vi "4145 Set GUI controls.vi"(0 "Simple/Advanced Checked?":bool, 5 "Panel Controls[]":refnum<vi>[](array[refnum]), 7 "X axis":bool, 9 "Y2 axis":bool, 11 "Is VAR 2 used?":bool) -> ()   [LabVIEW 2014]
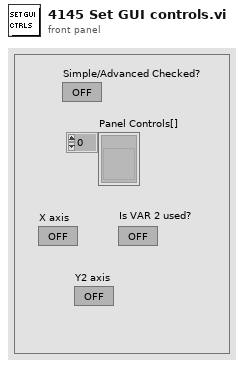
[diagram p1: front panel]
types:
  T1 = enum8{"Enabled", "Disabled", "Disabled and Grayed Out"}
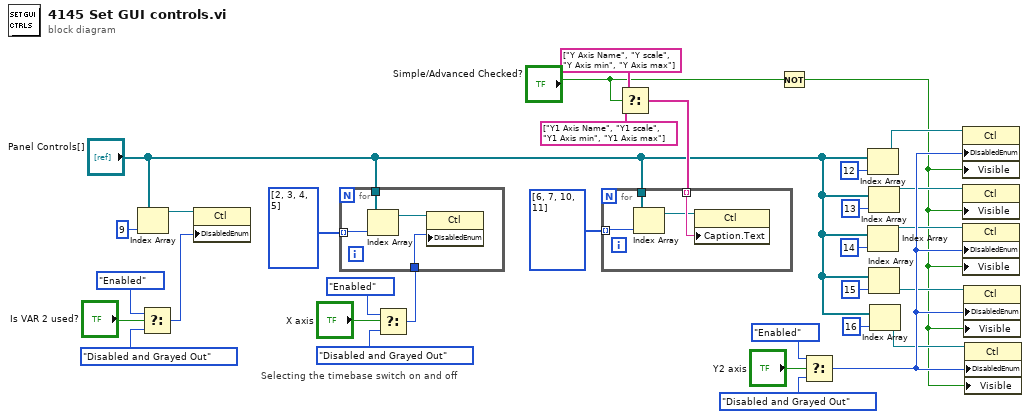
[diagram p0: block diagram]
diagram:
  # "Selecting the timebase switch on and off"
  n1 = Index Array(array="Panel Controls[]", index=9) -> (element=w5:refnum<vi>)
  n2 = Select(t=T1."Enabled" ("Disabled"), s="Is VAR 2 used?", f=T1."Disabled and Grayed Out" ("Disabled")) -> (s? t:f=w1:T1)
  n3 = property class="Ctl"(reference=w5, "DisabledEnum"=w1) -> ()  [unwired: 1 in, 2 out]
  n4 = Select(t=T1."Enabled" ("Disabled"), s="X axis", f=T1."Disabled and Grayed Out" ("Disabled")) -> (s? t:f=w11:T1)
  n5 = for {
    tunnel: w11 -> [w36]
    tunnel: i32[] [2, 3, 4, 5] -> [w35] mode=indexing
    tunnel: "Panel Controls[]" -> [w34]
    n6 = Index Array(array=w34, index=w35) -> (element=w33:refnum<vi>)
    n7 = property class="Ctl"(reference=w33, "DisabledEnum"=w36) -> ()  [unwired: 1 in, 2 out]
  }
  n8 = Select(t=string[] ["Y Axis Name", "Y scale", "Y Axis min", "Y Axis max"], s="Simple/Advanced Checked?", f=string[] ["Y1 Axis Name", "Y1 scale", "Y1 Axis min", "Y1 Axis max"]) -> (s? t:f=w8:string[])
  n9 = for {
    tunnel: i32[] [6, 7, 10, 11] -> [w40] mode=indexing
    tunnel: "Panel Controls[]" -> [w39]
    tunnel: w8 -> [w38] mode=indexing
    n10 = Index Array(array=w39, index=w40) -> (element=w37:refnum<vi>)
    n11 = property class="Ctl"(reference=w37, "Caption.Text"=w38) -> ()  [unwired: 1 in, 2 out]
  }
  n12 = Not(x="Simple/Advanced Checked?") -> (.not. x?=w12:bool)
  n13 = Select(t=T1."Enabled" ("Disabled"), s="Y2 axis", f=T1."Disabled and Grayed Out" ("Disabled")) -> (s? t:f=w32:T1)
  n14 = Index Array(array="Panel Controls[]", index=12) -> (element=w23:refnum<vi>)
  n15 = Index Array(array="Panel Controls[]", index=14) -> (element=w26:refnum<vi>)
  n16 = Index Array(array="Panel Controls[]", index=13) -> (element=w14:refnum<vi>)
  n17 = Index Array(array="Panel Controls[]", index=15) -> (element=w27:refnum<vi>)
  n18 = Index Array(array="Panel Controls[]", index=16) -> (element=w29:refnum<vi>)
  n19 = property class="Ctl"(reference=w23, "DisabledEnum"=w32, "Visible"=w12) -> ()  [unwired: 1 in, 2 out]
  n20 = property class="Ctl"(reference=w14, "Visible"=w12) -> ()  [unwired: 1 in, 2 out]
  n21 = property class="Ctl"(reference=w26, "DisabledEnum"=w32, "Visible"=w12) -> ()  [unwired: 1 in, 2 out]
  n22 = property class="Ctl"(reference=w27, "DisabledEnum"=w32, "Visible"=w12) -> ()  [unwired: 1 in, 2 out]
  n23 = property class="Ctl"(reference=w29, "DisabledEnum"=w32, "Visible"=w12) -> ()  [unwired: 1 in, 2 out]
